vi "Add Local Chassis from Config.vi"(8 "error in":errorcluster, 9 "Programming Mode":T1[](array[typedef]), 10 "Item Ref in":T2 format="%.0x", 11 "Modules":T3[](array[typedef])) -> (0 "error out":errorcluster)   [LabVIEW 2019, in "SEECD System Explorer.lvlib"]
uses:
  SEECD System Explorer.lvlib
  Type Defs/Host - Module.ctl
  Type Defs/IOV Container Contents.ctl
  <vilib>/NI VeriStand/Custom Device API/Custom Device Item Ref.ctl
  Type Defs/Slot Programming Mode.ctl
  Shared/Type Defs/Host - FPGAScanInterfaceMode.ctl
  Includes/Modules.lvlibp/RSI Module/Slot Settings.ctl
  Includes/Modules.lvlibp/RSI Module/Module Models.ctl
  Shared/Globals/Scan Engine GUIDs.vi
  Shared/Globals/Property Strings.vi
  Includes/Modules.lvlibp/RSI Module/Class Property Strings.vi
  <vilib>/NI VeriStand/Custom Device API/Set Item Property (U16).vi
  Shared/Globals/String Constants.vi
  Includes/Modules.lvlibp/RSI Module/RSI Module.lvclass
  <vilib>/NI VeriStand/Custom Device API/Custom Device API.lvlib
  Shared/SEECD Shared.lvlib
  Includes/Modules.lvlibp
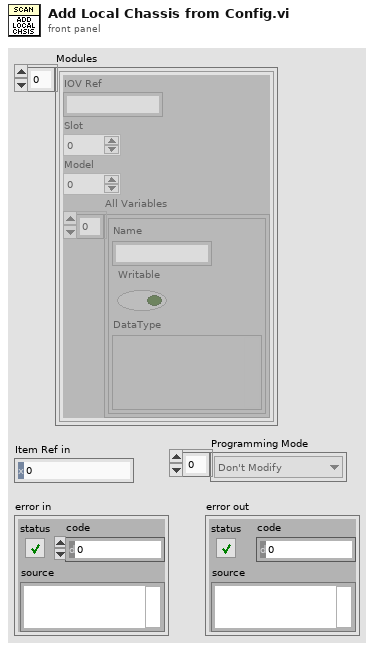
[diagram p1: front panel]
types:
  T1 = typedef "SEECD System Explorer.lvlib/Slot Programming Mode.ctl" = enum16{"Don't Modify", "Scan Engine", "LabVIEW FPGA", "NI-DAQmx"}
  T2 = typedef "Custom Device API.lvlib/Custom Device Item Ref.ctl" = u64
  T3 = typedef "SEECD System Explorer.lvlib/Host - Module.ctl" = cluster{"IOV Ref":string, "Slot":u32, "Model":u32, "All Variables":T4[]}
  T4 = typedef "SEECD System Explorer.lvlib/IOV Container Contents.ctl" = cluster{"Name":string, "Writable":bool, "DataType":variant}
  T5 = typedef "SEECD Shared.lvlib/Host - FPGAScanInterfaceMode.ctl" = enum16{"Use Current", "FPGA", "Scan Mode"}
  T6 = typedef "Modules.lvlibp/RSI Module.lvclass/Slot Settings.ctl" = cluster{"Slot":u32, "EtherCAT?":bool}
  T7 = typedef "Modules.lvlibp/RSI Module.lvclass/Module Models.ctl" = enum16{"Empty", "NI 9201", "NI 9203", "NI 9205", "NI 9206", "NI 9207", "NI 9208", "NI 9209", "NI 9210", "NI 9211", "NI 9212", "NI 9213", "NI 9214", "NI 9215", "NI 9216", "NI 9217", "NI 9219", "NI 9220", "NI 9221", "NI 9222", "NI 9223", "NI 9224", "NI 9225", "NI 9226", "NI 9227", "NI 9228", "NI 9229", "NI 9233", "NI 9234", "NI 9235", "NI 9236", "NI 9237", "NI 9239", "NI 9242", "NI 9244", "NI 9253", "NI 9263", "NI 9264", "NI 9265", "NI 9266", "NI 9269", "NI 9344", "NI 9350", "NI 9375", "NI 9401", "NI 9402", "NI 9403", "NI 9411", "NI 9421", "NI 9422", "NI 9423", "NI 9425", "NI 9426", "NI 9435", "NI 9436", "NI 9437", "NI 9472", "NI 9474", "NI 9475", "NI 9476", "NI 9477", "NI 9478", "NI 9481", "NI 9482", "NI 9485"}
  T8 = typedef "Modules.lvlibp/Custom Device API.lvlib/Custom Device Item Ref.ctl" = u64
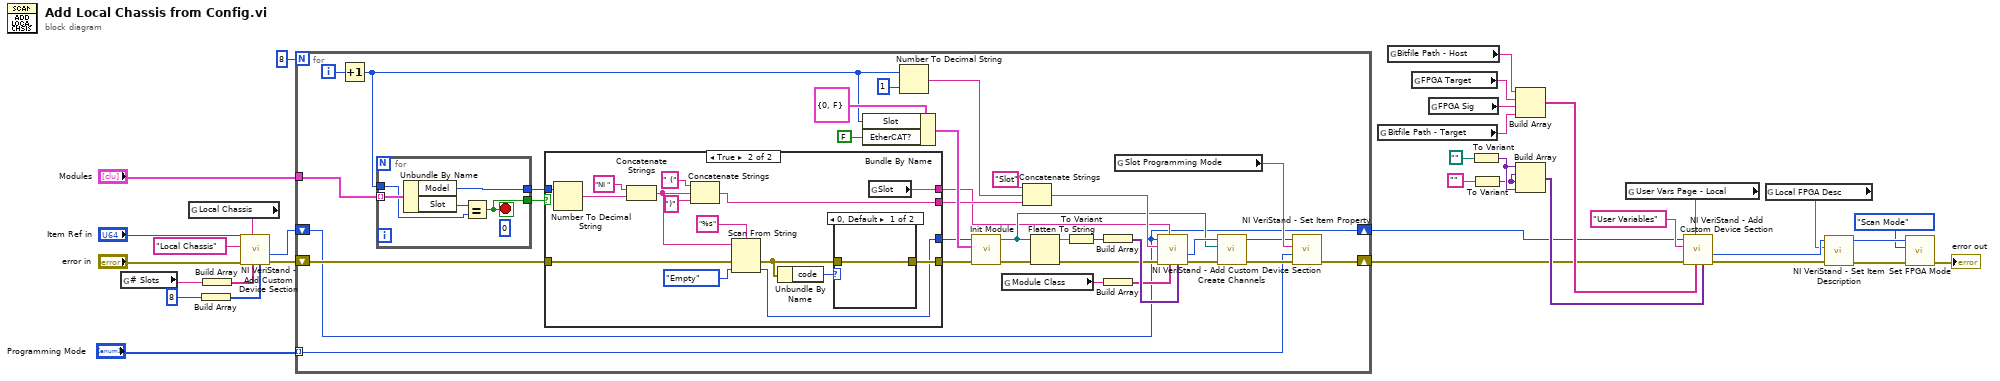
[diagram p0: block diagram]
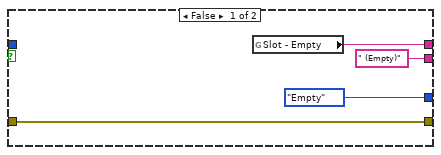
[diagram p2: hidden frame]
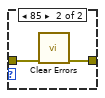
[diagram p3: hidden frame]
diagram:
  n1 = global read "Property Strings.vi" "# Slots"() -> (w6:string)
  n2 = global read "Scan Engine GUIDs.vi" "Local Chassis"() -> (w5:string)
  n3 = Build Array(8 ("# Slots")) -> (w8:i32[])
  n4 = Build Array(w6) -> (w7:string[])
  n5 = call <vilib>:"NI VeriStand - Add Custom Device Section.vi"("Property Values"=w8, "Property names"=w7, "GUID (Default Section)"=w5, "error in (no error)"="error in", "Section Name"="Local Chassis", "Parent Ref in"="Item Ref in") -> ("error out"=w11:errorcluster, "Section Ptr"=w13:T2)  [unwired: 2 in, 2 out]
  n6 = for {
    N: 8 -> [_]
    shift-right: [w38] -> w9
    shift-left: w11 -> [w47]
    shift-right: [w35] -> w10
    shift-left: w13 -> [w35]
    tunnel: "Modules" -> [w52]
    tunnel: "Programming Mode" -> [w36] mode=indexing
    i -> [w65]
    n7 = Increment(x=w65) -> (x+1=w51:i32)
    n8 = for {
      tunnel: w52 -> [w94] mode=indexing
      tunnel: w51 -> [w92]
      tunnel: [w91] -> w50
      tunnel: [w90] -> w45
      stop <- w91 stop-if-true
      (unwired) u32 0 ("Model")
      n9 = Unbundle By Name(w94) -> ("Model"=w90:u32, "Slot"=w93:u32)
      n10 = Equal?(x=w93, y=w92) -> (x = y?=w91:bool)
    }
    n11 = case shown="True" w50 {
      tunnel: [" (Empty)" ("Section Name") w73] -> w49
      tunnel: [Module_Models."Empty" ("Module") w80] -> w48
      tunnel: w47 -> [w69 w81]
      tunnel: [w69 w82] -> w46
      tunnel: w45 -> [_ w79]
      tunnel: [w68 w72] -> w41
      frame False {
        n12 = global read "Scan Engine GUIDs.vi" "Slot - Empty"() -> (w68:string)
      }
      frame True {
        n13 = Number To Decimal String(number=w79) -> (decimal integer string=w78:string)  [unwired: 1 in]
        n14 = Concatenate Strings("NI " ("string"), w78) -> (w76:string)
        n15 = Concatenate Strings(" (" ("string"), w76, ")" ("string")) -> (w73:string)
        n16 = Scan From String(format string="%s", input string=w76, error in=w81, default 1=Module_Models."Empty" ("Module")) -> (error out=w83:errorcluster, output 1=w80:T7)  [unwired: 1 in, 2 out]
        n17 = Unbundle By Name(w83) -> ("code"=w84:i32)
        n18 = case shown="0, Default" w84 {
          tunnel: [w87 w88] -> w82
          tunnel: w83 -> [w87 w89]
          frame 0, Default {
          }
          frame 85 {
            n19 = call <vilib>:"Clear Errors.vi"("error in (no error)"=w89) -> ("error out"=w88:errorcluster)  [unwired: 5 in, 1 out]
          }
        }
        n20 = global read "Scan Engine GUIDs.vi" "Slot"() -> (w72:string)
      }
    }
    n21 = Bundle By Name(cluster=T6 {"Slot"=0, "EtherCAT?"=FALSE} ("Slot Settings"), "Slot"=w51, "EtherCAT?"=FALSE) -> (w61:T6)
    n22 = Number To Decimal String(number=w51, width (-)=i16 1) -> (decimal integer string=w67:string)
    n23 = call "Init Module.vi"("error in (no error)"=w46, "Slot Settings"=w61, "Module Model"=w48) -> ("error out"=w56:errorcluster, "RSI Module out"=w42:refnum<class "RSI Module.lvclass">)  [unwired: 7 in]
    n24 = global read "Class Property Strings.vi" "Module Class"() -> (w54:string)
    n25 = Concatenate Strings("Slot" ("string"), w67, w49) -> (w64:string)
    n26 = Flatten To String(anything=w42, error in (no error)=w56) -> (data string=w57:string, error out=w55:errorcluster)  [unwired: 2 in, 1 out]
    n27 = To Variant(anything=w57) -> (Variant=w62:variant)
    n28 = Build Array(w62) -> (w63:variant[])
    n29 = Build Array(w54) -> (w58:string[])
    n30 = global read "Property Strings.vi" "Slot Programming Mode"() -> (w40:string)
    n31 = call <vilib>:"NI VeriStand - Add Custom Device Section.vi"("Property Values"=w63, "Property names"=w58, "GUID (Default Section)"=w41, "error in (no error)"=w55, "Section Name"=w64, "Parent Ref in"=w35) -> ("error out"=w43:errorcluster, "Section Ptr"=w44:T2)  [unwired: 2 in, 2 out]
    n32 = call-dynamic "Create Channels.vi"("error in (no error)"=w43, "RSI Module in"=w42, "Parent Ref in"=w44) -> ("error out"=w37:errorcluster, "Parent Ref out"=w39:T8)  [unwired: 6 in, 1 out]
    n33 = call-poly <vilib>:"NI VeriStand - Set Item Property.vi"("error in (no error)"=w37, "Value"=w36, "Property Name"=w40, "Item Ref in"=w39) -> ("error out"=w38:errorcluster)  [unwired: 5 in, 2 out]
  }
  n34 = global read "Property Strings.vi" "Bitfile Path - Target"() -> (w19:string)
  n35 = global read "Property Strings.vi" "Bitfile Path - Host"() -> (w22:string)
  n36 = global read "Property Strings.vi" "FPGA Target"() -> (w21:string)
  n37 = global read "Property Strings.vi" "FPGA Sig"() -> (w20:string)
  n38 = To Variant(anything=path "") -> (Variant=w18:variant)
  n39 = To Variant(anything="") -> (Variant=w16:variant)
  n40 = Build Array(w22, w21, w20, w19) -> (w24:string[])
  n41 = Build Array(w18, w16, w16, w18) -> (w25:variant[])
  n42 = global read "Scan Engine GUIDs.vi" "User Vars Page - Local"() -> (w26:string)
  n43 = call <vilib>:"NI VeriStand - Add Custom Device Section.vi"("Property Values"=w25, "Property names"=w24, "GUID (Default Section)"=w26, "error in (no error)"=w9, "Section Name"="User Variables", "Parent Ref in"=w10) -> ("error out"=w30:errorcluster, "Section Ptr"=w29:T2)  [unwired: 2 in, 2 out]
  n44 = global read "String Constants.vi" "Local FPGA Desc"() -> (w27:string)
  n45 = call <vilib>:"NI VeriStand - Set Item Description.vi"("error in (no error)"=w30, "Description"=w27, "Item Ref in"=w29) -> ("error out"=w32:errorcluster, "Item Ref out"=w34:T2)  [unwired: 6 in, 1 out]
  n46 = call "Set FPGA Mode.vi"("error in (no error)"=w32, "FPGAScanInterfaceMode"=Host_-_FPGAScanInterfaceMode."Scan Mode", "Item Ref in"=w34) -> ("error out"=→"error out":errorcluster)  [unwired: 7 in, 1 out]
